vi "Check for Hot Pixel Location Mismatch (U8).vi"(8 "error in (no error)":errorcluster, 9 "SS3 Hot Pixel Mismatch Detection":bool, 11 "Array in":u8[][](array[numeric])) -> (0 "error out":errorcluster, 3 "Array (dup)":u8[][](array[numeric]))   [LabVIEW 2021]
uses:
  64ae88dd-af2e-4fb4-b9b8-bc1122bb5c19.vi
  0e7b5a21-2934-42ff-966f-67b280e6b2d5.vi
  7a266268-73c8-4a63-8716-e157ce5b39d7.vi
  7a266268-73c8-4a63-8716-e157ce5b39d7.vi/d4db2432-cc9c-482c-8957-dac855435ef6.vi
  7a266268-73c8-4a63-8716-e157ce5b39d7.vi/86fbf154-bd7b-49a2-8ab2-a837b2a95f24.vi
  7a266268-73c8-4a63-8716-e157ce5b39d7.vi/3b95b01e-1ec2-4565-bcd9-7606a5281010.vi
  7a266268-73c8-4a63-8716-e157ce5b39d7.vi/96a08935-737a-44b2-979c-a81d56408f7e.vi
  7a266268-73c8-4a63-8716-e157ce5b39d7.vi/d4db2432-cc9c-482c-8957-dac855435ef6.vi/6eaecd13-6e48-4772-a921-b51ebdf84d88.vi
  7a266268-73c8-4a63-8716-e157ce5b39d7.vi/d4db2432-cc9c-482c-8957-dac855435ef6.vi/d2d5f2b7-06f4-47f6-971c-049c3fdbb653.vi
  7a266268-73c8-4a63-8716-e157ce5b39d7.vi/3b95b01e-1ec2-4565-bcd9-7606a5281010.vi/6eaecd13-6e48-4772-a921-b51ebdf84d88.vi
  7a266268-73c8-4a63-8716-e157ce5b39d7.vi/3b95b01e-1ec2-4565-bcd9-7606a5281010.vi/d2d5f2b7-06f4-47f6-971c-049c3fdbb653.vi
  7a266268-73c8-4a63-8716-e157ce5b39d7.vi/96a08935-737a-44b2-979c-a81d56408f7e.vi/6eaecd13-6e48-4772-a921-b51ebdf84d88.vi
  7a266268-73c8-4a63-8716-e157ce5b39d7.vi/96a08935-737a-44b2-979c-a81d56408f7e.vi/d2d5f2b7-06f4-47f6-971c-049c3fdbb653.vi
  <vilib>/Utility/error.llb/Error Cluster From Error Code.vi
  <vilib>/Comparison/Less/Less Functor/Less Functor.lvclass
  <vilib>/ErrorRing/Error Ring.xnode
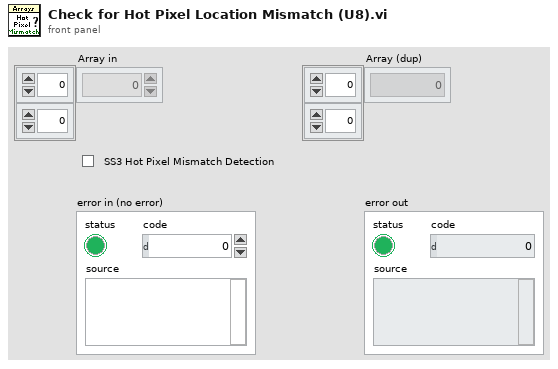
[diagram p1: front panel]
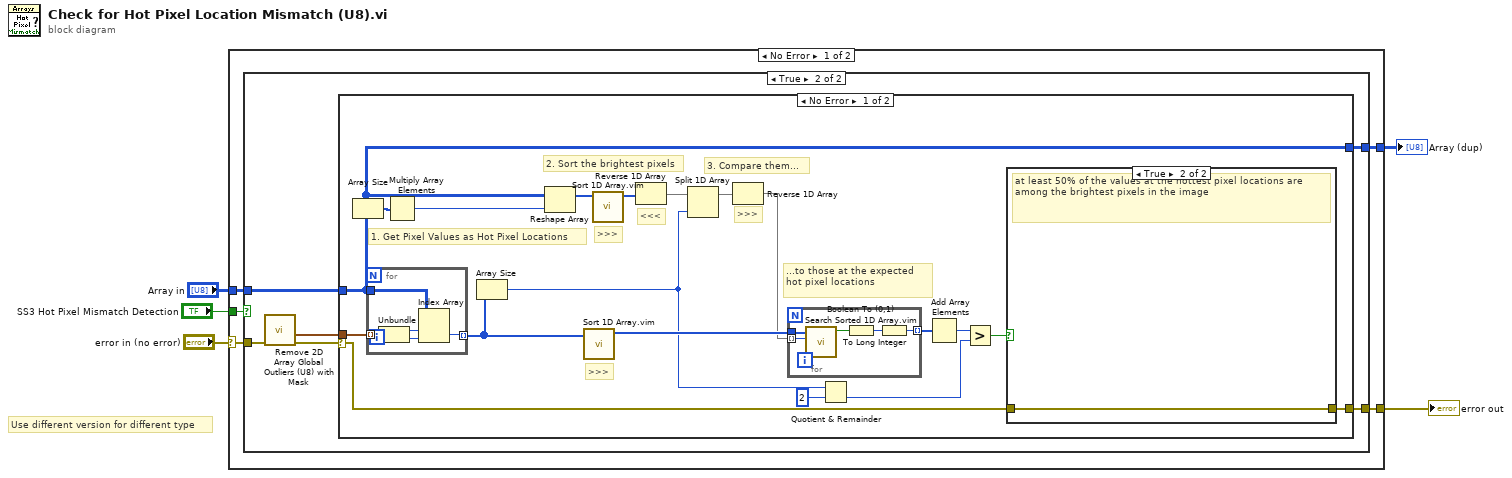
[diagram p0: block diagram]
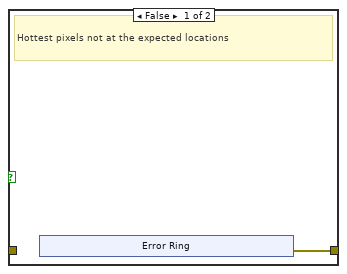
[diagram p3: hidden frame]
diagram:
  # "Use different version for different type"
  n1 = case shown="No Error" "error in (no error)" {
    selector: "error in (no error)" -> [w8 w56]
    tunnel: "Array in" -> [w10 w55]
    tunnel: [w9 w56] -> w4
    tunnel: "SS3 Hot Pixel Mismatch Detection" -> [w7 _]
    tunnel: [w6 w55] -> w1
    frame No Error {
      n2 = case shown="True" w7 {
        tunnel: w10 -> [w11 w16]
        tunnel: [w12 w14] -> w9
        tunnel: w8 -> [w12 w15]
        tunnel: [w11 w13] -> w6
        frame False {
        }
        frame True {
          n3 = call "Remove 2D Array Global Outliers (U8) with Mask.vi"("Error In"=w15) -> ("Error Out"=w17:errorcluster, "Hot Pixel Locations"=w18:cluster{"Numeric":i32, "Numeric":i32}[])  [unwired: 7 in, 2 out]
          n4 = case shown="No Error" w17 {
            selector: w17 -> [w36 _]
            tunnel: w18 -> [w37 _]
            tunnel: w16 -> [w27 w54]
            tunnel: [w30 _] -> w14
            tunnel: [w27 w54] -> w13
            frame No Error {
              # ">>>"
              # ">>>"
              # "<<<"
              # ">>>"
              # "...to those at the expected hot pixel locations"
              # "3. Compare them..."
              # "2. Sort the brightest pixels"
              # "1. Get Pixel Values as Hot Pixel Locations"
              n5 = Array Size(array=w27) -> (size(s)=w34:i32[])
              n6 = for {
                tunnel: w37 -> [w53] mode=indexing
                tunnel: [w49] -> w28 mode=indexing
                tunnel: w27 -> [w52]
                n7 = Unbundle(w53) -> ("Numeric"=w51:i32, "Numeric"=w50:i32)
                n8 = Index Array(array=w52, index (row)=w51, index (col)=w50) -> (element=w49:u8)
              }
              n9 = Multiply Array Elements(1:w34) -> (0:w33:i32)
              n10 = Array Size(array=w28) -> (size(s)=w21:i32)
              n11 = Reshape Array(w27, w33) -> (w35:u8[])
              n12 = call "Sort 1D Array.vim"("unsorted array"=w28) -> ("sorted array"=w26:u8[])  [unwired: 10 in]
              n13 = call "Sort 1D Array.vim"("unsorted array"=w35) -> ("sorted array"=w32:u8[])  [unwired: 10 in]
              n14 = Reverse 1D Array(array=w32) -> (reversed array=w31:u8[])
              n15 = Split 1D Array(array=w31, index=w21) -> (first subarray=w29:u8[])  [unwired: 1 out]
              n16 = Reverse 1D Array(array=w29) -> (reversed array=w25:u8[])
              n17 = for {
                tunnel: w26 -> [w48]
                tunnel: w25 -> [w47] mode=indexing
                tunnel: [w44] -> w24 mode=indexing
                n18 = call "Search Sorted 1D Array.vim"("element"=w47, "sorted 1D array"=w48) -> ("found?"=w46:bool)  [unwired: 8 in, 1 out]
                n19 = Boolean To (0,1)(Boolean=w46) -> (0, 1=w45:i16)
                n20 = To Long Integer(number=w45) -> (32bit integer=w44:i32)
              }
              n21 = Quotient & Remainder(x=w21, y=2) -> (floor(x/y)=w22:i32)  [unwired: 1 out]
              n22 = Add Array Elements(numeric array=w24) -> (sum=w23:i32)
              n23 = Greater?(x=w23, y=w22) -> (0:w19:bool)
              n24 = case shown="True" w19 {
                tunnel: w36 -> [_ w43]
                tunnel: [w38 w43] -> w30
                frame False {
                  # "Hottest pixels not at the expected locations"
                  n25 = xnode "Error Ring"() -> ("error out"=w38:errorcluster)
                }
                frame True {
                  # "at least 50% of the values at the hottest pixel locations are among the brightest pixels in the image"
                }
              }
            }
            frame Error {
              # "Not Hot Pixel Map defined: ignore"
            }
          }
        }
      }
    }
    frame Error {
    }
  }
  "error out" <- w4
  "Array (dup)" <- w1
